vi "FTW-Container-Value-Boolean.vi"(0 "FTW-Container In":refnum<class "FTW-Container.lvclass">, 11 "error in":errorcluster) -> (4 "FTW-Container Out":refnum<class "FTW-Container.lvclass">, 8 "Value":bool, 15 "error out":errorcluster)   [LabVIEW 2015, in "FTW-Container.lvclass"]
uses:
  FTW-Container.lvclass
  FTW-Container.lvclass/FTW-Container.ctl
  <vilib>/Utility/Data Type/NI_Data Type.lvlib
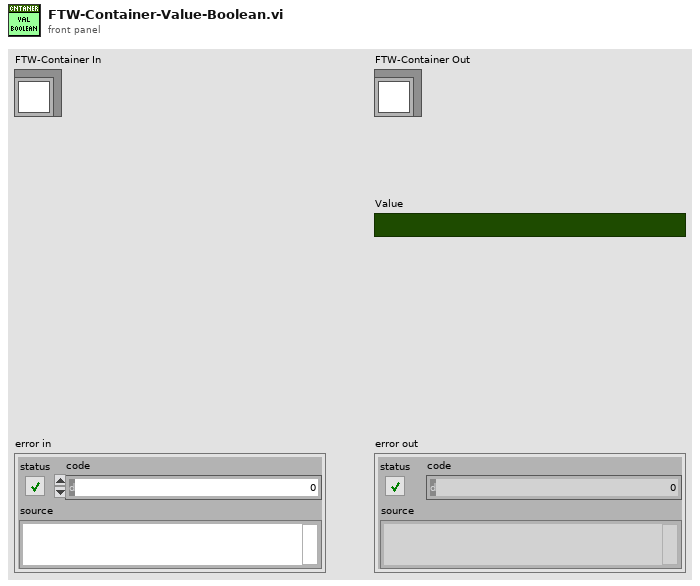
[diagram p1: front panel]
types:
  T1 = typedef "NI_Data Type.lvlib/Data Type.ctl" = enum8{"Invalid Type", "Void", "I8", "I16", "I32", "I64", "U8", "U16", "U32", "U64", "Single Float", "Double Float", "Extended Float", "Single Complex", "Double Complex", "Extended Complex", "Enum U8", "Enum U16", "Enum U32", "Enum U64", "Single Float With Unit", "Double Float With Unit", "Extended Float With Unit", "Single Complex with Unit", "Double Complex with Unit", "Extended Complex with Unit", "Boolean", "String", "Path", "Picture", "Tag", "Array", "Cluster", "Variant", "LV Variant", "Waveform", "Timestamp", "Digital Waveform", "Digital Data", "ExpressData", "Refnum", "External Data", "VI", "Poly VI", "LabVIEW Class Instance", "Fixed Point"}
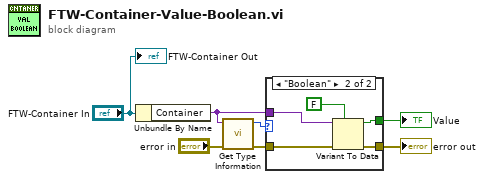
[diagram p0: block diagram]
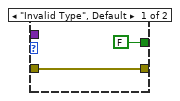
[diagram p2: hidden frame]
diagram:
  n1 = Unbundle By Name("FTW-Container In") -> ("Container"=w1:variant)
  n2 = call <vilib>:"Get Type Information.vi"("error in (no error)"="error in", "Variant"=w1) -> ("error out"=w6:errorcluster, "Type"=w3:T1)  [unwired: 5 in, 3 out]
  n3 = case shown="\"Boolean\"" w3 {
    tunnel: w6 -> [w9 w14]
    tunnel: [w9 w13] -> w4
    tunnel: [FALSE w11] -> w2
    tunnel: w1 -> [_ w12]
    frame "Invalid Type", Default {
    }
    frame "Boolean" {
      n4 = Variant To Data(error in=w14, type=FALSE, Variant=w12) -> (data=w11:bool, error out=w13:errorcluster)
    }
  }
  "error out" <- w4
  "Value" <- w2
  "FTW-Container Out" <- "FTW-Container In"
